vi "SVPO Integration (1 CH DBL WDT).vi"(6 "reset filters":bool, 7 "desired base units for length":i32(ring)=-1 items=["no change"=-1, "m"=0, "mm"=2, "microns"=3, "in"=1, "mils"=5], 9 "highpass cutoff frequency [Hz]":dbl=1.0 format="%.2f", 11 "scaled signal [EU]":waveform(dbl)) -> (3 "integrated signal [EU*s]":waveform(dbl))   [LabVIEW 2017, in "SoundVib_Integration.lvlib"]
doc: "Converts acceleration to velocity or velocity to displacement using a time-domain waveform as the input. Wire data to the <B>scaled signal [EU]</B> input to determine the polymorphic instance to use or manually select the instance. This VI performs Single Integration only. You can pass the integrated signal [EU*s] output to the scaled signal [EU] input of second call to this VI to perform double integration."
uses:
  <vilib>/addons/Sound and Vibration/svt_Integration/SoundVib_Integration.lvlib
  <vilib>/addons/Sound and Vibration/svt_Integration/SVPO Integration (1 CH DBL Array) with IC.vi
  <vilib>/addons/Sound and Vibration/svt_Integration/subVIs/svl_Integration Units.vi
  <vilib>/addons/Sound and Vibration/svt_Integration/subVIs/svl_Apply Highpass Filter with IC.vi
  <vilib>/addons/Sound and Vibration/svt_Integration/subVIs/svl_Low Pass [Order 1] No State.vi
  <vilib>/addons/Sound and Vibration/svt_Integration/subVIs/svl_Design HighPass Filter.vi
  <vilib>/addons/Sound and Vibration/svt_Integration/subVIs/svl_RC Filter Coefficients.vi
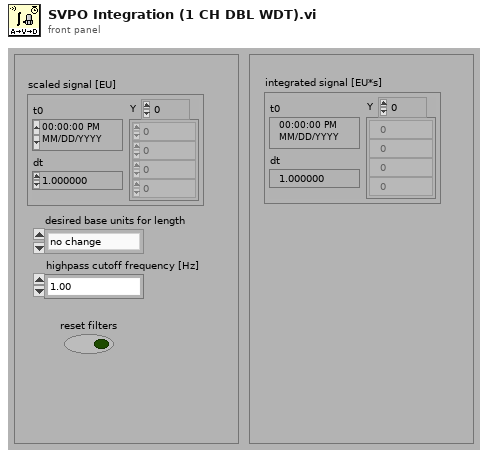
[diagram p1: front panel]
types:
  T1 = typedef "svc_Integration State.ctl" = cluster{"filter coefficents":cluster{"integration filter coefficients":cluster{"beta":dbl, "gamma":dbl, "alpha":dbl}, "highpass filter coefficients":cluster{"filter structure":enum32{"IIR 2nd Order", "IIR 4th Order"}, "Reverse Coefficients":dbl[], "Forward Coefficients":dbl[]}}, "filter state":cluster{"initial integration fiter state":cluster{"x(n-1) state":dbl, "y(n-1) state":dbl, "x(n-2) state":dbl, "y(n-2) state":dbl}, "initial highpass filter state":dbl[]}}
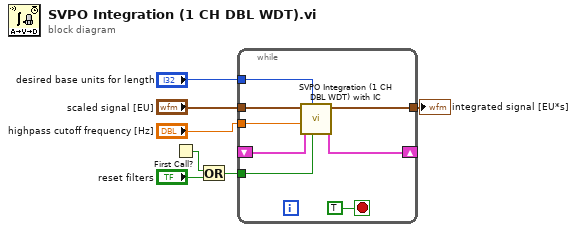
[diagram p0: block diagram]
diagram:
  n1 = First Call?() -> (First Call?: T/F=w4:bool)
  n2 = Or(x=w4, y="reset filters") -> (x .or. y?=w2:bool)
  n3 = while {
    tunnel: "scaled signal [EU]" -> [w15]
    tunnel: "highpass cutoff frequency [Hz]" -> [w14]
    tunnel: [w13] -> w5
    tunnel: w2 -> [w9]
    shift-right: [w11] -> _
    shift-left: _ -> [w12]
    tunnel: "desired base units for length" -> [w8]
    stop <- TRUE stop-if-true
    n4 = call <vilib>:"SVPO Integration (1 CH DBL WDT) with IC.vi"("reset filters"=w9, "desired base units for length"=w8, "initial conditions"=w12, "highpass cutoff frequency [Hz]"=w14, "scaled signal [EU]"=w15) -> ("final conditions"=w11:T1, "integrated signal [EU*s]"=w13:waveform(dbl))  [unwired: 5 in]
  }
  "integrated signal [EU*s]" <- w5
